vi "Hyphenation.vi"(8 "error in":errorcluster, 11 "Word":string) -> (0 "error out":errorcluster, 3 "Hyphenated":string[](array[string]))   [LabVIEW 2020]
doc: "Odd numbers indicate that hyphenation is allowed at that index"
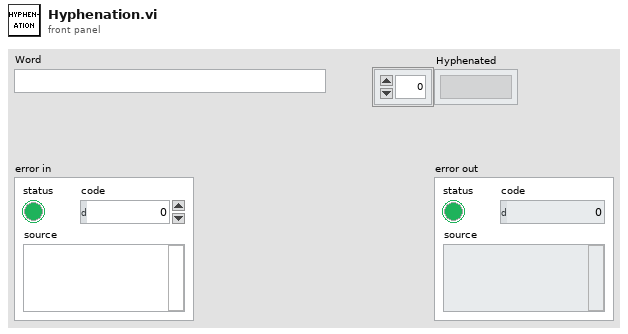
[diagram p1: front panel]
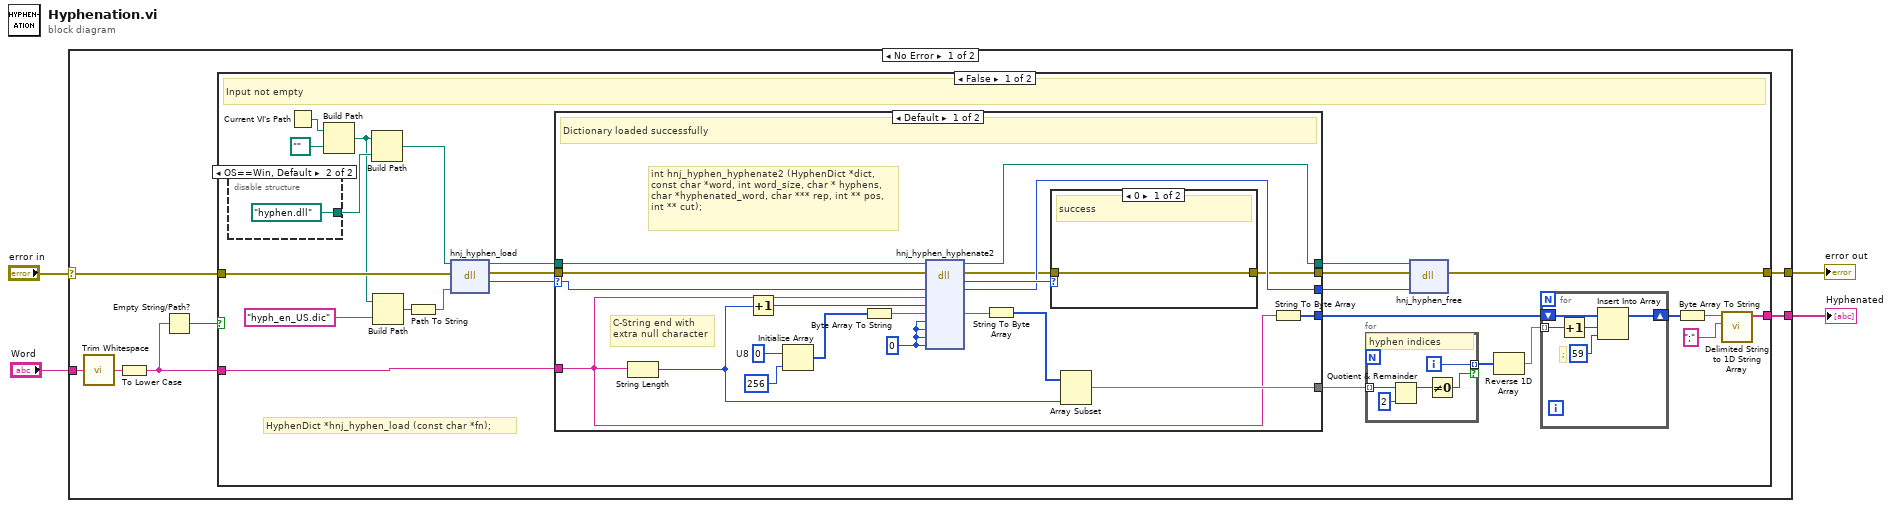
[diagram p0: block diagram]
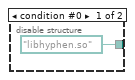
[diagram p2: hidden frame]
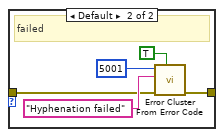
[diagram p3: hidden frame]
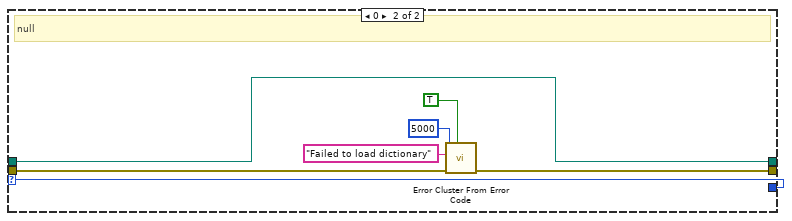
[diagram p4: hidden frame]
diagram:
  n1 = case shown="No Error" "error in" {
    selector: "error in" -> [w11 w83]
    tunnel: [w10 w83] -> w3
    tunnel: "Word" -> [w9 _]
    tunnel: [w5 _] -> w1
    frame No Error {
      n2 = call <vilib>:"Trim Whitespace.vi"("string"=w9) -> ("trimmed string"=w7:string)  [unwired: 1 in]
      n3 = To Lower Case(string=w7) -> (all lower case string=w6:string)
      n4 = Empty String/Path?(string/path=w6) -> (empty?=w8:bool)
      n5 = case shown="False" w8 {
        tunnel: w11 -> [w36 w82]
        tunnel: [w32 w82] -> w10
        tunnel: w6 -> [w30 _]
        tunnel: [w14 _] -> w5
        frame False {
          # "HyphenDict *hnj_hyphen_load (const char *fn);"
          # "Input not empty"
          n6 = disable-structure shown="OS==Win, Default" {
            disable-tunnel: [path "libhyphen.so" ("path in") path "hyphen.dll" ("path in")] -> w25
            frame condition #0 {
            }
            frame condition #1 (active) {
            }
          }
          n7 = Current VI's Path() -> (path=w27:path)
          n8 = Build Path(base path=w27, name or relative path=path "..") -> (appended path=w23:path)
          n9 = Build Path(base path=w23, name or relative path=w25) -> (appended path=w24:path)
          n10 = Build Path(base path=w23, name or relative path="hyph_en_US.dic") -> (appended path=w21:path)
          n11 = Path To String(path=w21) -> (string=w20:string)
          n12 = dll-call lib="?" fn="hnj_hyphen_load"(path in=w24, error in=w36, ".dic"=w20) -> (path out=w31:path, error out=w35:errorcluster, "return type"=w34:u64)  [unwired: 2 in]
          n13 = case shown="Default" w34 {
            selector: w34 -> [w66 w75]
            tunnel: w35 -> [w68 w81]
            tunnel: [w61 w80] -> w33
            tunnel: w31 -> [w67 w76]
            tunnel: w30 -> [w50 _]
            tunnel: [w64 w75] -> w29
            tunnel: [w63 w76] -> w28
            tunnel: [w51 _] -> w19
            tunnel: [w49 _] -> w13
            frame Default {
              w58 = u64 0
              w59 = u8 0  # U8
              # "C-String end with\nextra null character"
              # "int hnj_hyphen_hyphenate2 (HyphenDict *dict, const char *word, int word_size, char * hyphens, char *hyphenated_word, char *** rep, int ** pos, int ** cut);"
              # "Dictionary loaded successfully"
              n14 = String Length(string=w50) -> (length=w52:i32)
              n15 = Increment(x=w52) -> (x+1=w56:i32)
              n16 = Initialize Array(w59, 256 ("y")) -> (w60:u8[])
              n17 = Byte Array To String(unsigned byte array=w60) -> (string=w57:string)
              n18 = dll-call lib="?" fn="hnj_hyphen_hyphenate2"(path in=w67, error in=w68, "dict"=w66, "word"=w50, "word_size"=w56, "hyphens"=w57, "hyphenated_word"=w58, "rep"=w58, "pos"=w58, "cut"=w58) -> (path out=w63:path, error out=w62:errorcluster, "return type"=w65:i32, "dict"=w64:u64, "hyphens"=w54:string)  [unwired: 7 in]
              n19 = String To Byte Array(string=w54) -> (unsigned byte array=w53:u8[])
              n20 = case shown="0" w65 {
                tunnel: w62 -> [w69 w72]
                tunnel: [w69 w71] -> w61
                frame 0 {
                  # "success"
                }
                frame Default {
                  # "failed"
                  n21 = call <vilib>:"Error Cluster From Error Code.vi"("show call chain? (False)"=TRUE, "error in (no error)"=w72, "error message (\"\")"="Hyphenation failed" ("error message (\"\")"), "error code (0)"=5001) -> ("error out"=w71:errorcluster)  [unwired: 5 in]
                }
              }
              n22 = Array Subset(array=w53, length=w52) -> (w51:u8[])  [unwired: 1 in]
              n23 = String To Byte Array(string=w50) -> (unsigned byte array=w49:u8[])
            }
            frame 0 {
              # "null"
              n24 = call <vilib>:"Error Cluster From Error Code.vi"("show call chain? (False)"=TRUE, "error in (no error)"=w81, "error message (\"\")"="Failed to load dictionary" ("error message (\"\")"), "error code (0)"=5000) -> ("error out"=w80:errorcluster)  [unwired: 5 in]
            }
          }
          n25 = for {
            tunnel: w19 -> [w46] mode=indexing
            tunnel: [w43] -> w18 mode=indexing if=w42
            i -> [w43]
            # "hyphen indices"
            n26 = Quotient & Remainder(x=w46, y=2) -> (x-y*floor(x/y)=w44:i32)  [unwired: 1 out]
            n27 = Not Equal To 0?(x=w44) -> (x != 0?=w42:bool)
          }
          n28 = dll-call lib="?" fn="hnj_hyphen_free"(path in=w28, error in=w33, "dic"=w29) -> (error out=w32:errorcluster)  [unwired: 3 in, 1 out]
          n29 = Reverse 1D Array(array=w18) -> (reversed array=w12:i32[])
          n30 = for {
            shift-right: [w39] -> w17
            shift-left: w13 -> [w41]
            tunnel: w12 -> [w38] mode=indexing
            # ";"
            n31 = Increment(x=w38) -> (x+1=w37:i32)
            n32 = Insert Into Array(array=w41, index=w37, new element=u8 59 ("new element/subarray")) -> (w39:u8[])
          }
          n33 = Byte Array To String(unsigned byte array=w17) -> (string=w16:string)
          n34 = call <vilib>:"Delimited String to 1D String Array.vi"("delimiter"=";", "delimited string"=w16) -> ("string array"=w14:string[])  [unwired: 9 in]
        }
        frame True {
          # "Input empty"
        }
      }
    }
    frame Error {
    }
  }
  "error out" <- w3
  "Hyphenated" <- w1
